vi "translate to peaks data spreadsheet.vi"(7 "peaks data":T1) -> (8 "peaks data":dbl[][](array[numeric]))   [LabVIEW 2009]
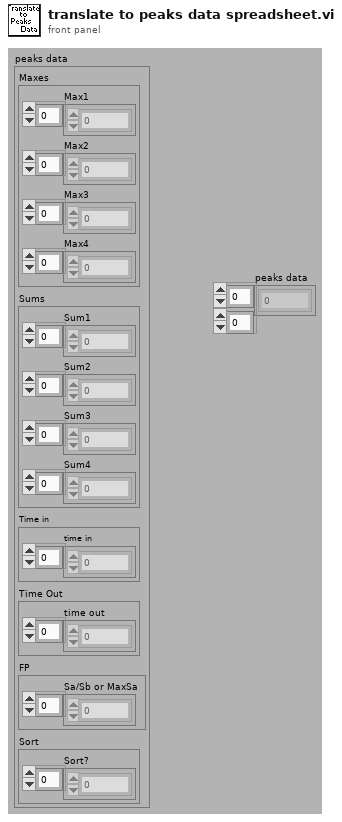
[diagram p1: front panel]
types:
  T1 = cluster{"Maxes":cluster{"Max1":dbl[], "Max2":dbl[], "Max3":dbl[], "Max4":dbl[]}, "Sums":cluster{"Sum1":dbl[], "Sum2":dbl[], "Sum3":dbl[], "Sum4":dbl[]}, "Time in":cluster{"time in":dbl[]}, "Time Out":cluster{"time out":dbl[]}, "FP":cluster{"Sa/Sb or MaxSa":dbl[]}, "Sort":cluster{"Sort?":dbl[]}}
  T2 = cluster{"Max1":dbl[], "Max2":dbl[], "Max3":dbl[], "Max4":dbl[]}
  T3 = cluster{"Sum1":dbl[], "Sum2":dbl[], "Sum3":dbl[], "Sum4":dbl[]}
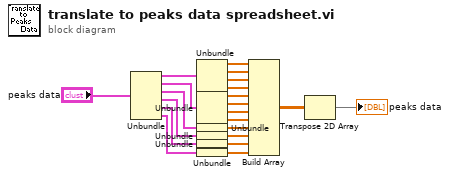
[diagram p0: block diagram]
diagram:
  n1 = Unbundle("peaks data") -> ("Maxes"=w21:T2, "Sums"=w20:T3, "Time in"=w19:cluster{"time in":dbl[]}, "Time Out"=w18:cluster{"time out":dbl[]}, "FP"=w17:cluster{"Sa/Sb or MaxSa":dbl[]}, "Sort"=w1:cluster{"Sort?":dbl[]})
  n2 = Unbundle(w21) -> ("Max1"=w16:dbl[], "Max2"=w15:dbl[], "Max3"=w14:dbl[], "Max4"=w13:dbl[])
  n3 = Unbundle(w20) -> ("Sum1"=w12:dbl[], "Sum2"=w11:dbl[], "Sum3"=w10:dbl[], "Sum4"=w9:dbl[])
  n4 = Unbundle(w19) -> ("time in"=w8:dbl[])
  n5 = Unbundle(w18) -> ("time out"=w7:dbl[])
  n6 = Unbundle(w17) -> ("Sa/Sb or MaxSa"=w6:dbl[])
  n7 = Unbundle(w1) -> ("Sort?"=w2:dbl[])
  n8 = Build Array(w16, w15, w14, w13, w12, w11, w10, w9, w8, w7, w6, w2) -> (w5:dbl[][])
  n9 = Transpose 2D Array(2D array=w5) -> (transposed array=→"peaks data":dbl[][])
